vi "CheesyDrive.vi"(5 "Quick Stop Alpha":dbl=0.1, 6 "Max Output":dbl=1.0, 7 "QuickStopThreshold":dbl=0.2, 9 "Quick Turn":bool, 10 "Turn":dbl, 11 "Throttle":dbl) -> (2 "Right Motor Value":dbl, 3 "Left Motor Value":dbl)   [LabVIEW 2018]
panel:
  in  "Turn Scalar":dbl
  in  "Square Inputs":bool=TRUE
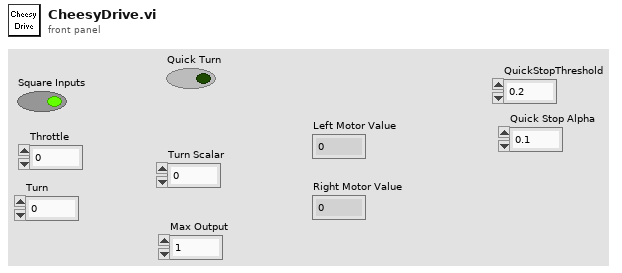
[diagram p1: front panel]
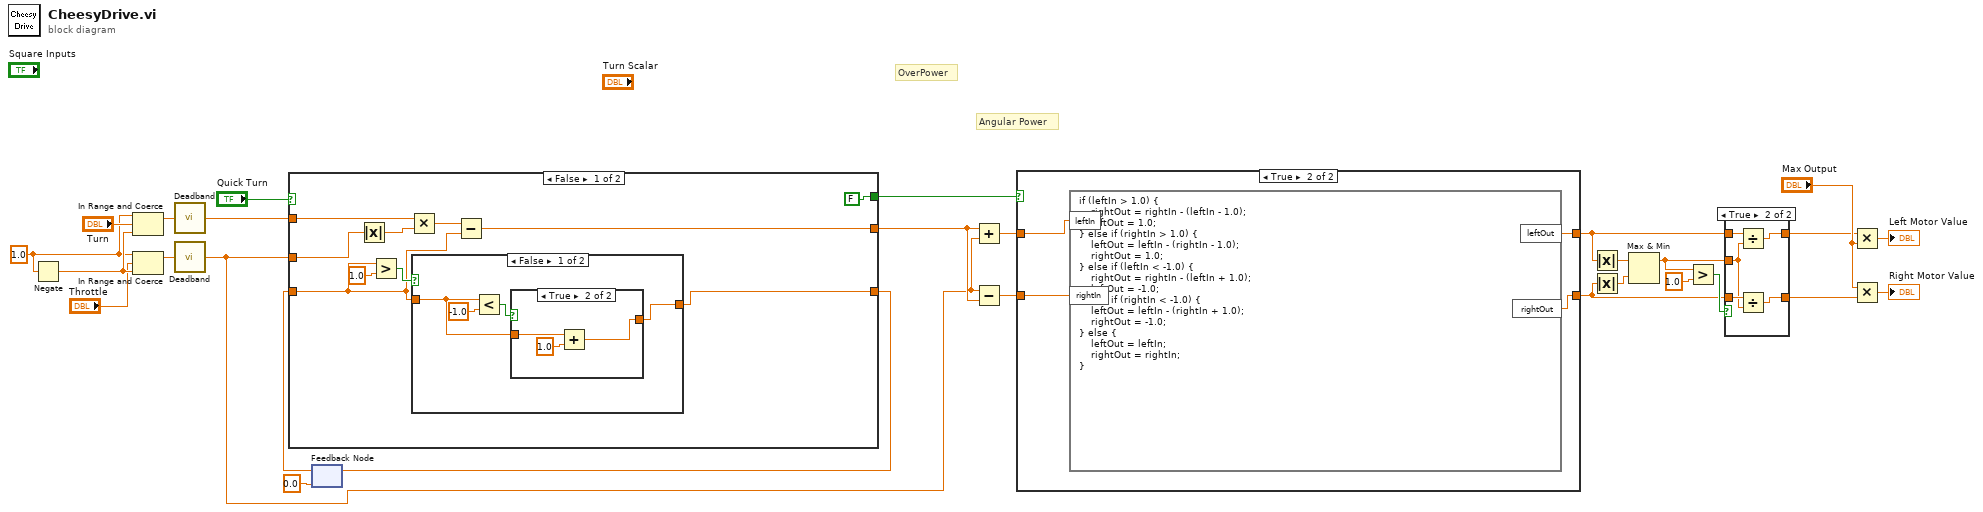
[diagram p0: block diagram]
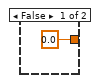
[diagram p4: hidden frame]
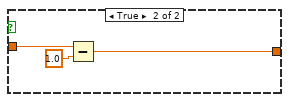
[diagram p5: hidden frame]
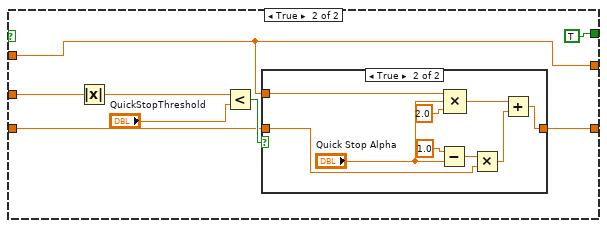
[diagram p6: hidden frame]
diagram:
  w24 = 1.0 ("x")
  # "OverPower"
  # "Angular Power"
  n1 = Negate(x=w24) -> (-x=w27:dbl)
  n2 = In Range and Coerce(upper limit=w24, x="Turn", lower limit=w27) -> (coerced(x)=w25:dbl)  [unwired: 1 out]
  n3 = In Range and Coerce(upper limit=w24, x="Throttle", lower limit=w27) -> (coerced(x)=w26:dbl)  [unwired: 1 out]
  n4 = call "Deadband.vi"("Value"=w25) -> ("Output"=w22:dbl)  [unwired: 3 in]
  n5 = call "Deadband.vi"("Value"=w26) -> ("Output"=w1:dbl)  [unwired: 3 in]
  n6 = feedback #1(0.0 ("x")) -> (w19:dbl)
  n7 = case shown="False" "Quick Turn" {
    tunnel: [FALSE TRUE] -> w16
    tunnel: w1 -> [w38 w54]
    tunnel: w22 -> [w36 w51]
    tunnel: [w30 w52] -> w21
    tunnel: w19 -> [w31 w53]
    tunnel: [w33 w51] -> w17
    frame False {
      n8 = Absolute Value(x=w38) -> (abs(x)=w37:dbl)
      n9 = Greater?(x=w31, y=1.0) -> (0:w32:bool)
      n10 = Multiply(x=w36, y=w37) -> (x*y=w35:dbl)
      n11 = case shown="False" w32 {
        tunnel: w31 -> [w40 w49]
        tunnel: [w39 w47] -> w30
        frame False {
          n12 = Less?(x=w40, y=-1.0) -> (x < y?=w41:bool)
          n13 = case shown="True" w41 {
            tunnel: w40 -> [_ w46]
            tunnel: [0.0 w44] -> w39
            frame False {
            }
            frame True {
              n14 = Add(x=w46, y=1.0) -> (x+y=w44:dbl)
            }
          }
        }
        frame True {
          n15 = Subtract(x=w49, y=1.0) -> (x-y=w47:dbl)
        }
      }
      n16 = Subtract(x=w35, y=w31) -> (x-y=w33:dbl)
    }
    frame True {
      n17 = Absolute Value(x=w54) -> (abs(x)=w57:dbl)
      n18 = Less?(x=w57, y="QuickStopThreshold") -> (x < y?=w55:bool)
      n19 = case shown="True" w55 {
        tunnel: w53 -> [w58 w65]
        tunnel: w51 -> [_ w61]
        tunnel: [w58 w59] -> w52
        frame False {
        }
        frame True {
          n20 = Subtract(x=1.0, y="Quick Stop Alpha") -> (x-y=w66:dbl)
          n21 = Compound Arithmetic op=MULTIPLY(w61, "Quick Stop Alpha", 2.0 ("value")) -> (w63:dbl)
          n22 = Multiply(x=w66, y=w65) -> (x*y=w64:dbl)
          n23 = Add(x=w63, y=w64) -> (x+y=w59:dbl)
        }
      }
    }
  }
  n24 = feedback-in #1(w21) -> ()
  n25 = Add(x=w17, y=w1) -> (x+y=w15:dbl)
  n26 = Subtract(x=w1, y=w17) -> (x-y=w14:dbl)
  n27 = case shown="True" w16 {
    tunnel: w15 -> [w69 w73]
    tunnel: [w69 w70] -> w10
    tunnel: [w68 w71] -> w8
    tunnel: w14 -> [w68 w72]
    frame False {
    }
    frame True {
      n28 = formula code="if (leftIn > 1.0) {\n    rightOut = rightIn - (leftIn - 1.0);\n    leftOut = 1.0;\n} else if (rightIn > 1.0) {\n    leftOut = leftIn - (rightIn - 1.0);\n    rightOut = 1.0;\n} else if (leftIn < -1.0) {\n    rightOut = rightIn - (leftIn + 1.0);\n    leftOut = -1.0;\n} else if (rightIn < -1.0) {\n    leftOut = leftIn - (rightIn + 1.0);\n    rightOut = -1.0;\n} else {\n    leftOut = leftIn;\n    rightOut = rightIn;\n}"("leftIn"=w73, "rightIn"=w72) -> ("leftOut"=w70:dbl, "rightOut"=w71:dbl)
    }
  }
  n29 = Absolute Value(x=w10) -> (abs(x)=w12:dbl)
  n30 = Absolute Value(x=w8) -> (abs(x)=w9:dbl)
  n31 = Max & Min(x=w12, y=w9) -> (max(x,y)=w7:dbl)  [unwired: 1 out]
  n32 = Greater?(x=w7, y=1.0) -> (0:w11:bool)
  n33 = case shown="True" w11 {
    tunnel: w10 -> [w75 w80]
    tunnel: w8 -> [w74 w79]
    tunnel: w7 -> [_ w78]
    tunnel: [w74 w77] -> w5
    tunnel: [w75 w76] -> w4
    frame False {
    }
    frame True {
      n34 = Divide(x=w80, y=w78) -> (x/y=w76:dbl)
      n35 = Divide(x=w79, y=w78) -> (x/y=w77:dbl)
    }
  }
  n36 = Multiply(x=w4, y="Max Output") -> (x*y=→"Left Motor Value":dbl)
  n37 = Multiply(x="Max Output", y=w5) -> (x*y=→"Right Motor Value":dbl)
